vi "UserVars-Parse Vector Function.vi"(0 "Expr in":string, 11 "error in (no error)":errorcluster) -> (4 "Expr out":string, 15 "error out":errorcluster)   [LabVIEW 2020]
uses:
  Math VIs/LinSpace (start-stop-step).vi
  <vilib>/regexp/Match Regular Expression.xnode
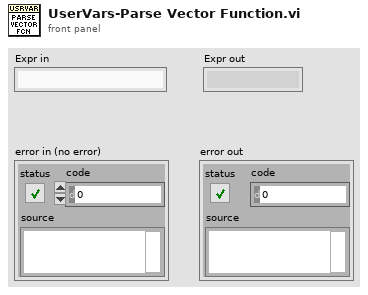
[diagram p1: front panel]
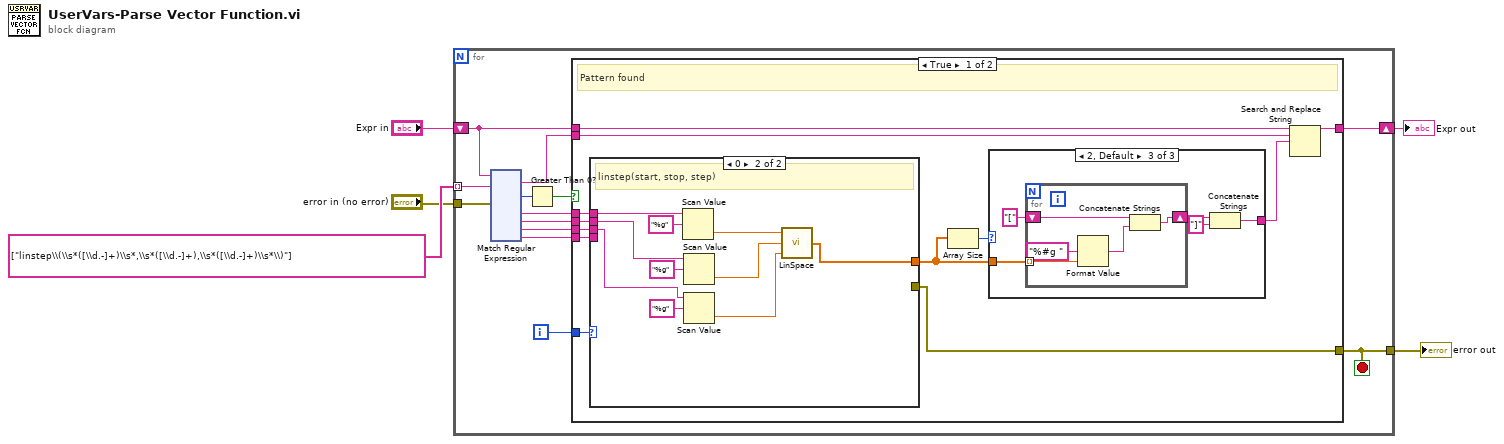
[diagram p0: block diagram]
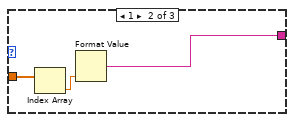
[diagram p3: hidden frame]
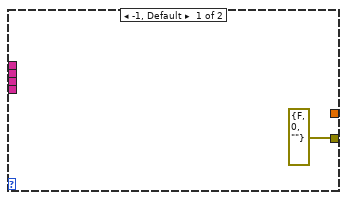
[diagram p4: hidden frame]
diagram:
  n1 = for {
    shift-right: [w15] -> w2
    shift-left: "Expr in" -> [w16]
    tunnel: string[] ["linstep\\(\\s*([\\d.-]+)\\s*,\\s*([\\d.-]+),\\s*([\\d.-]+)\\s*\\)"] ("String") -> [w7] mode=indexing
    tunnel: "error in (no error)" -> [w18]
    tunnel: [w8] -> w1
    i -> [w10]
    stop <- w8 stop-if-true
    n2 = xnode "Match Regular Expression"("input string"=w16, "regular expression"=w7, "error in"=w18) -> ("whole match"=w14:string, "offset past match"=w17:i32, "submatch 1"=w13:string, "submatch 2"=w12:string, "submatch 3"=w9:string, "submatch 4"=w6:string)  [unwired: 3 in, 3 out]
    n3 = Greater Than 0?(x=w17) -> (x > 0?=w11:bool)
    n4 = case shown="True" w11 {
      tunnel: w16 -> [w25 w55]
      tunnel: [w22 w55] -> w15
      tunnel: w14 -> [w24 _]
      tunnel: w13 -> [w29 _]
      tunnel: w12 -> [w28 _]
      tunnel: w10 -> [w30 _]
      tunnel: w9 -> [w27 _]
      tunnel: [w26 _] -> w8
      tunnel: w6 -> [w21 _]
      frame True {
        # "Pattern found"
        n5 = case shown="0" w30 {
          tunnel: w29 -> [_ w54]
          tunnel: w28 -> [_ w51]
          tunnel: [_ w45] -> w19
          tunnel: w27 -> [_ w49]
          tunnel: [errorcluster {"status"=FALSE, "code"=0, "source"=""} ("error constant") _] -> w26
          tunnel: w21 -> [_ _]
          frame -1, Default {
          }
          frame 0 {
            # "linstep(start, stop, step)"
            n6 = Scan Value(string=w54, format string="%g") -> (value=w48:dbl)  [unwired: 1 in, 1 out]
            n7 = Scan Value(string=w51, format string="%g") -> (value=w47:dbl)  [unwired: 1 in, 1 out]
            n8 = Scan Value(string=w49, format string="%g") -> (value=w46:dbl)  [unwired: 1 in, 1 out]
            n9 = call-poly "LinSpace.vi"("Step"=w46, "Stop"=w47, "Start"=w48) -> ("Array"=w45:dbl[])  [unwired: 1 in, 1 out]
          }
        }
        n10 = Array Size(array=w19) -> (size(s)=w20:i32)
        n11 = case shown="2, Default" w20 {
          tunnel: [_ w33 w34] -> w23
          tunnel: w19 -> [_ w32 w38]
          frame 0 {
          }
          frame 1 {
            n12 = Index Array(array=w32) -> (element=w31:dbl)  [unwired: 1 in]
            n13 = Format Value(value (0)=w31) -> (output string=w33:string)  [unwired: 2 in]
          }
          frame 2, Default {
            n14 = for {
              tunnel: w38 -> [w43] mode=indexing
              shift-right: [w41] -> w36
              shift-left: "[" -> [w40]
              n15 = Format Value(format string="%#g ", value (0)=w43) -> (output string=w39:string)  [unwired: 1 in]
              n16 = Concatenate Strings(w40, w39) -> (w41:string)
            }
            n17 = Concatenate Strings(w36, "]" ("string")) -> (w34:string)
          }
        }
        n18 = Search and Replace String(input string=w25, search string=w24, replace string=w23) -> (result string=w22:string)  [unwired: 5 in, 3 out]
      }
      frame False {
      }
    }
  }
  "error out" <- w1
  "Expr out" <- w2
